vi "FisherPaykel GET Visa.vi"(8 "Error In":errorcluster) -> (0 "Error Out":errorcluster, 1 "Use GEA Inverter Output":bool, 2 "Disable Serial COM (Debug ONLY) OUT":bool, 3 "VISA Output":refnum<visa-resource-name>, 4 "Machine ID Output":string, 6 "Inverter ID Output":string)   [LabVIEW 2016]
uses:
  Trunk/Utility/LabVIEW GEA2 Toolkit v1.0.0.0/library/GEA2_Toolkit.lvlib
panel:
  in  "Tab Control":enum32{"F&P Inverter", "GEA Inverter", "Debug"}(tab)
  in  "Discover Motor Interfaces":bool
  out "Motor Controllers Found":refnum<visa-resource-name>[](array[refnum])
  in  "Motor Controller Reference":refnum<visa-resource-name>
  out "Message":string
  in  "Inverter ID":string(combo)
  in  "Machine ID":string(combo)
  out "Detected Green Beans":string[](array[string])
  in  "Use GEA Inverter":bool
  in  "Discover GE Interfaces":bool
  in  "Disable Serial COM (Debug ONLY)":bool
  in  "Complete":bool
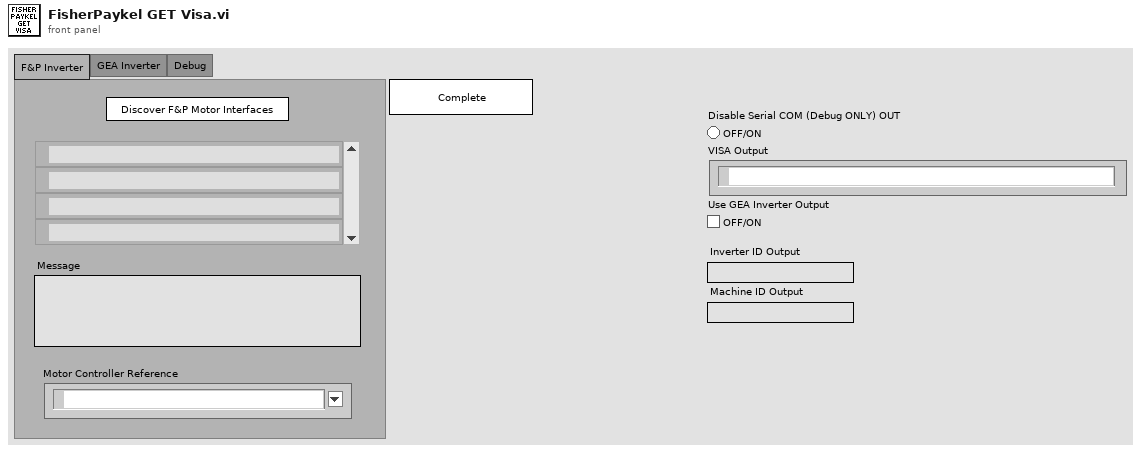
[diagram p1: front panel]
types:
  T1 = enum8{"Enabled", "Disabled", "Disabled and Grayed Out"}
  T2 = enum32{"invalid app kind", "Development System", "Run Time System", "Student Edition", "Embedded LabVIEW", "Evaluation", "Custom"}
  T3 = enum32{"Invalid", "Standard", "Closed", "Hidden", "Minimized", "Maximized"}
  T4 = cluster{"Core":cluster{"Current VI Reference":refnum<vi>, "Close Panel on Exit?":bool}, "Your Boolean data":bool, "Your string data":string}
  T5 = cluster{"Current VI Reference":refnum<vi>, "Close Panel on Exit?":bool}
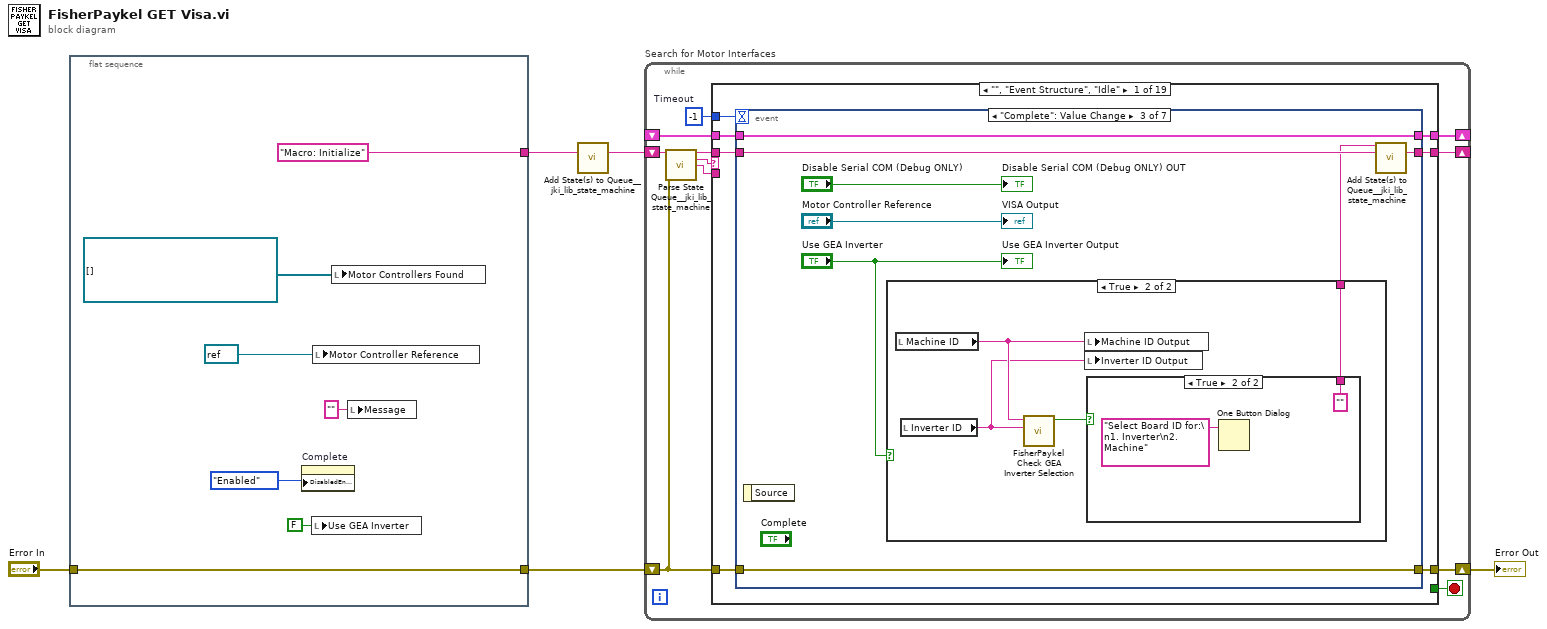
[diagram p0: block diagram]
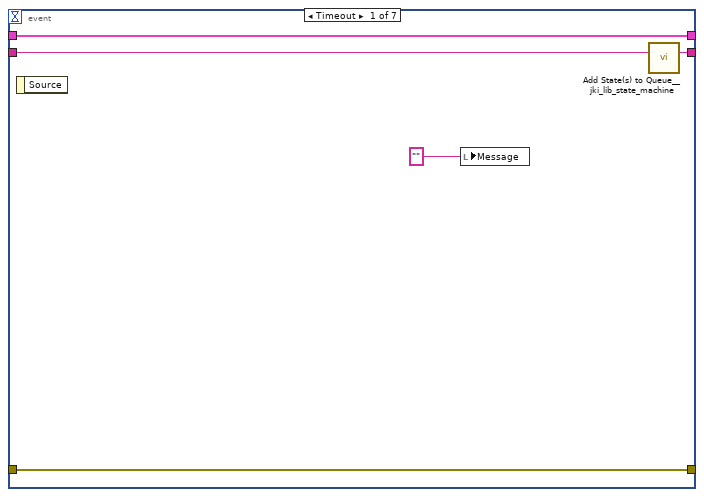
[diagram p2: hidden frame]
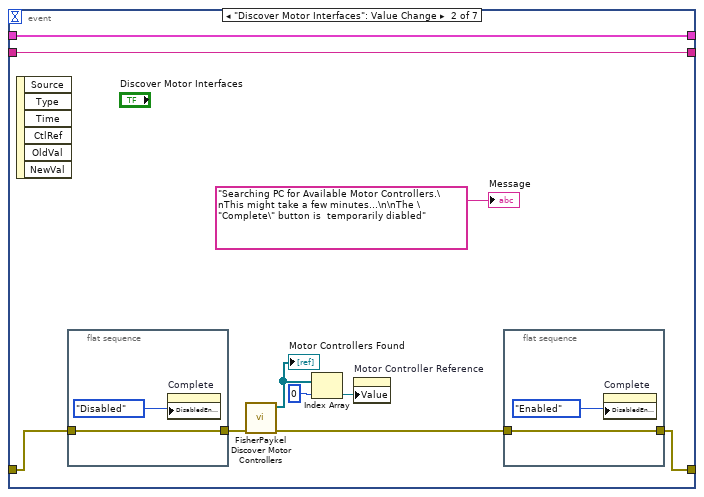
[diagram p3: hidden frame]
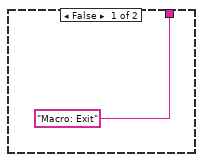
[diagram p4: hidden frame]
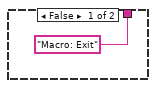
[diagram p5: hidden frame]
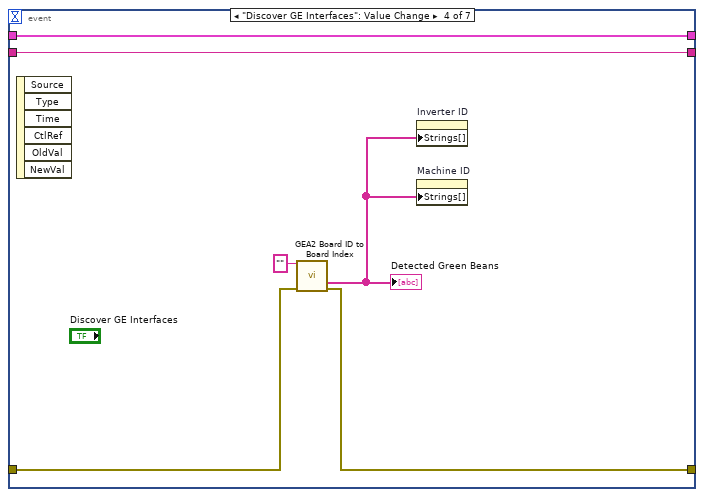
[diagram p6: hidden frame]
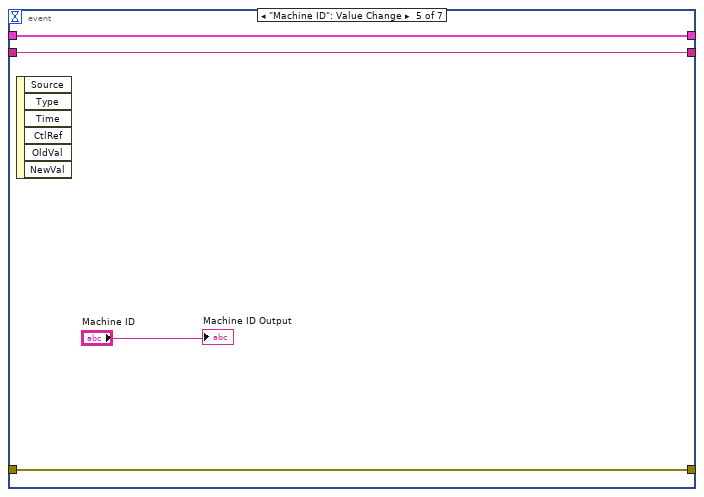
[diagram p7: hidden frame]
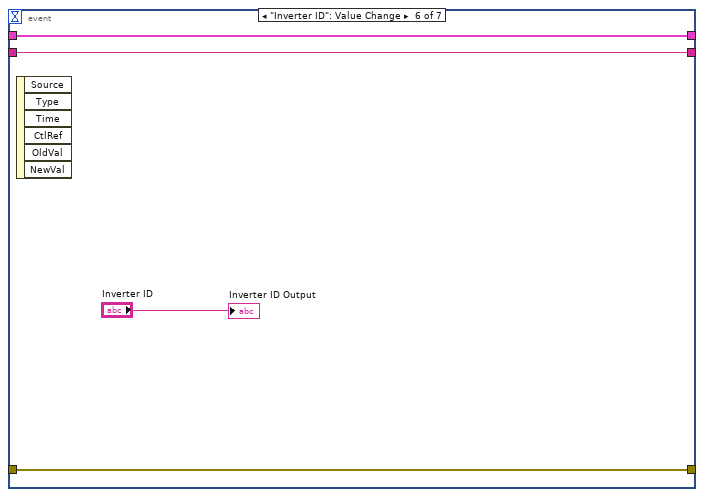
[diagram p8: hidden frame]
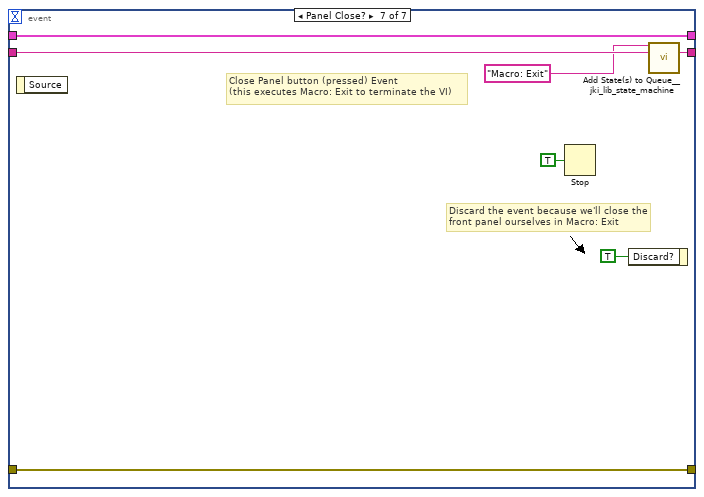
[diagram p9: hidden frame]
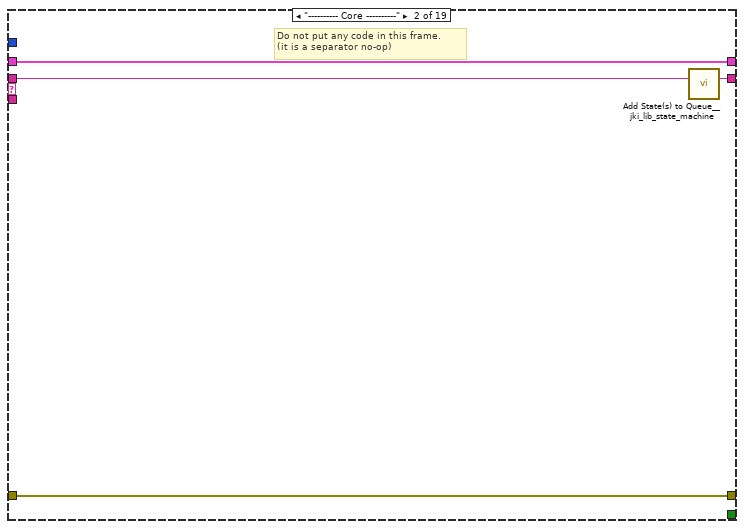
[diagram p10: hidden frame]
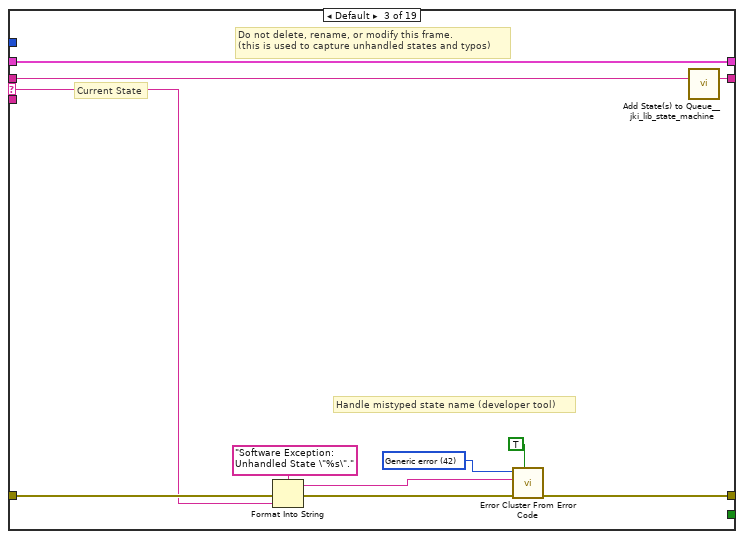
[diagram p11: hidden frame]
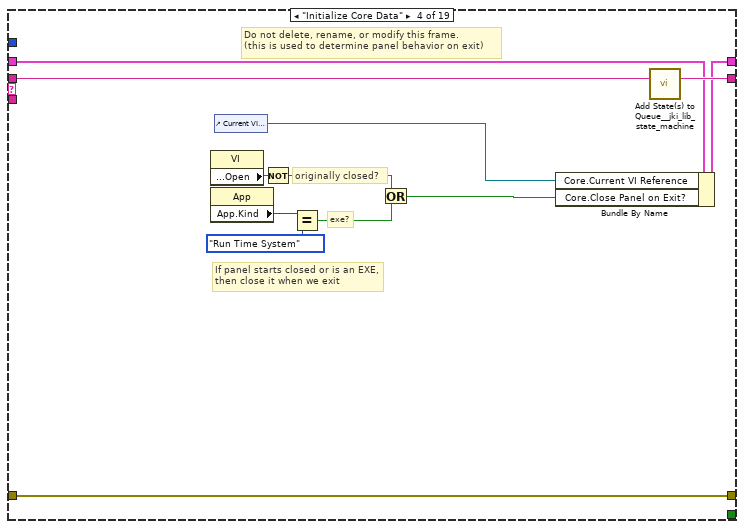
[diagram p12: hidden frame]
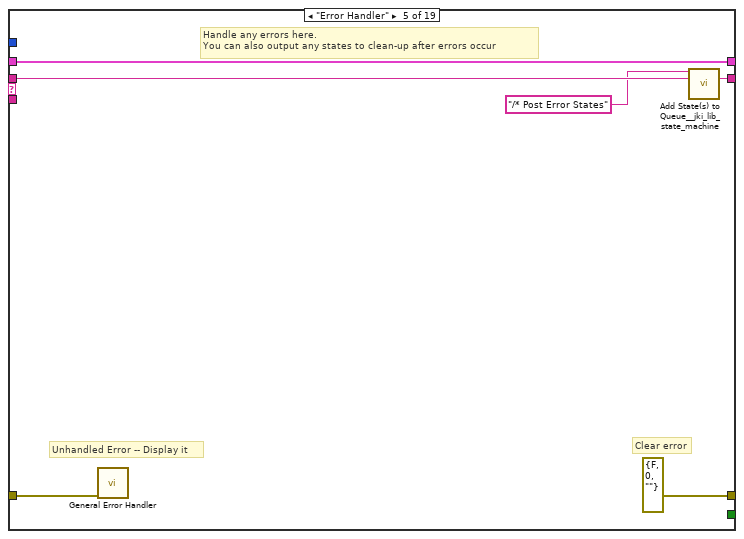
[diagram p13: hidden frame]
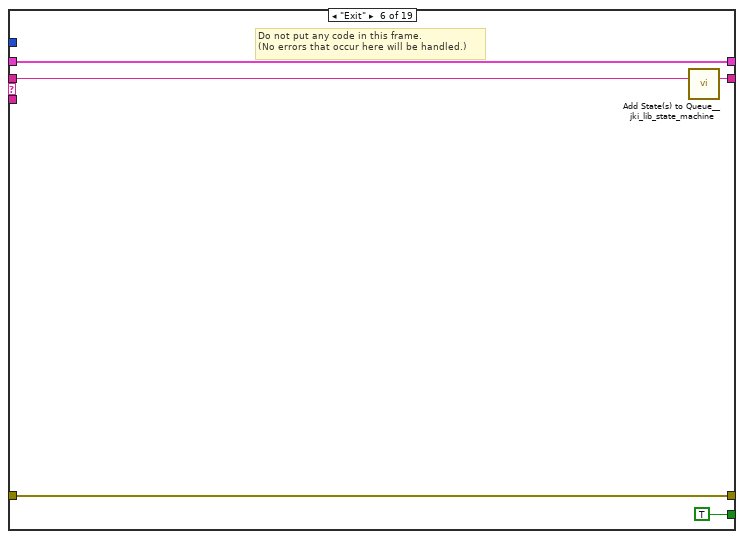
[diagram p14: hidden frame]
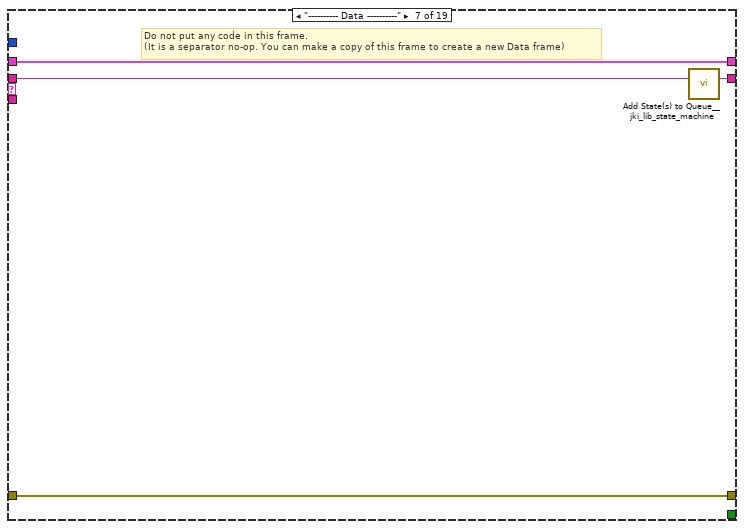
[diagram p15: hidden frame]
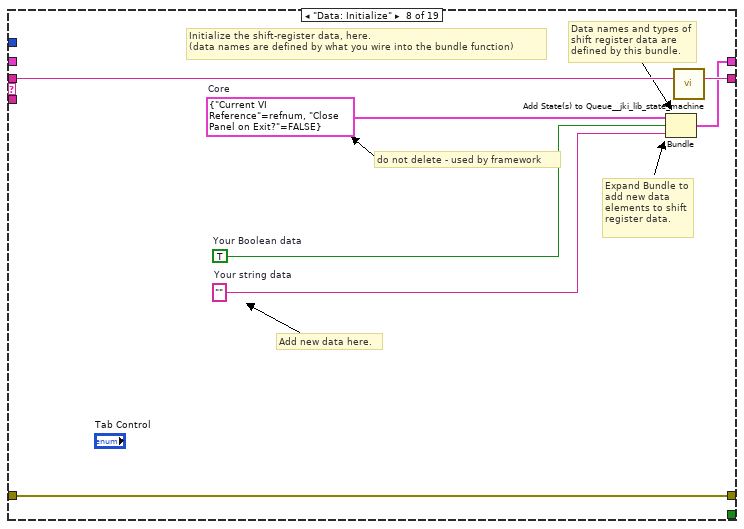
[diagram p16: hidden frame]
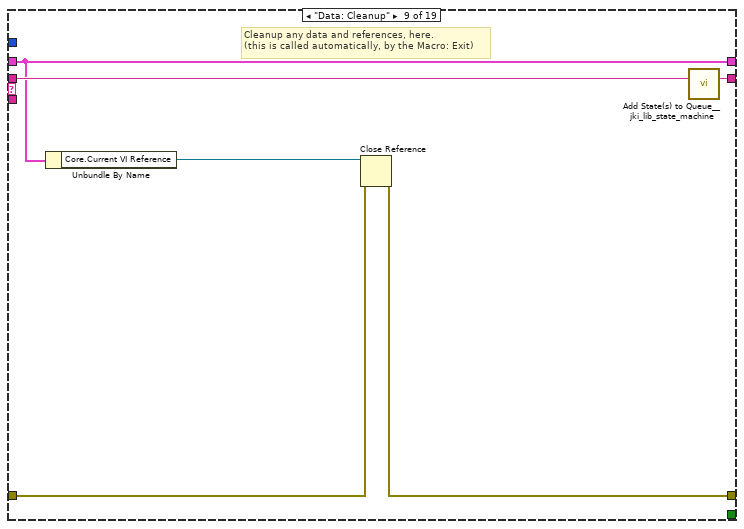
[diagram p17: hidden frame]
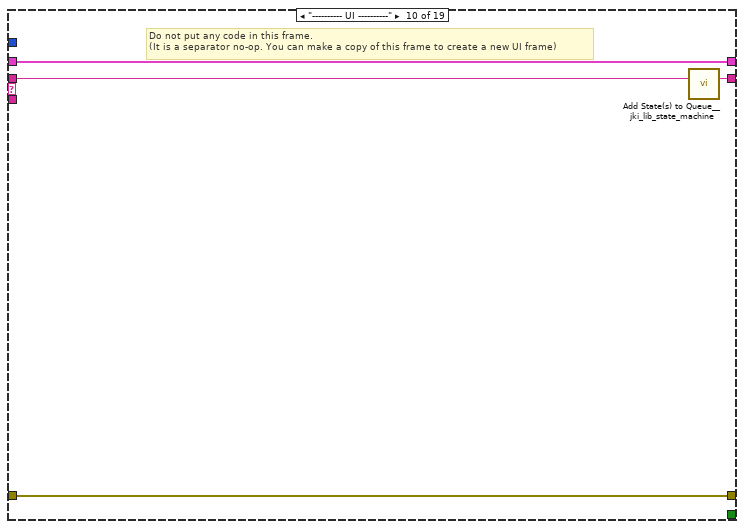
[diagram p18: hidden frame]
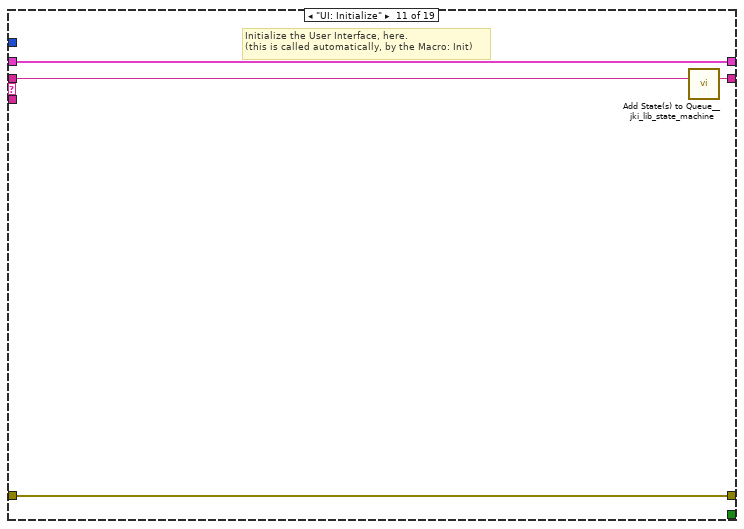
[diagram p19: hidden frame]
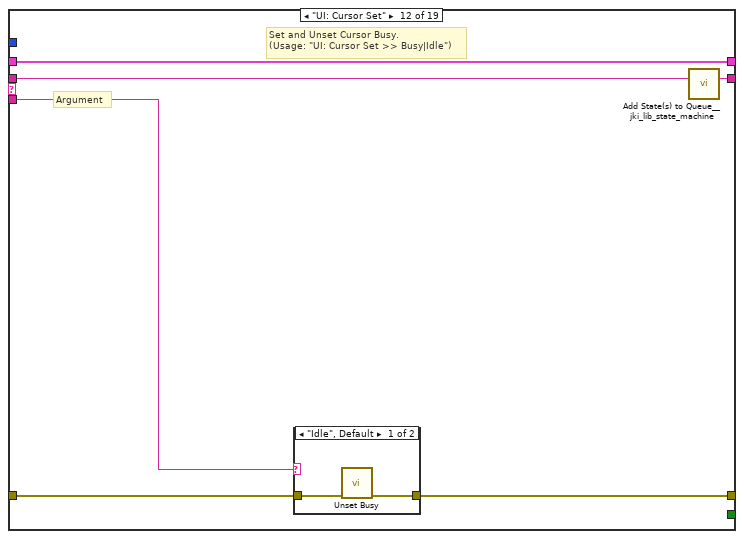
[diagram p20: hidden frame]
diagram:
  n1 = flat-sequence {
    tunnel: ["Macro: Initialize"] -> w4
    tunnel: [w7] -> w1
    tunnel: "Error In" -> [w7]
    frame #0 {
      n2 = property on="Complete" class="Bool"("DisabledEnum"=T1."Enabled" ("Disabled")) -> ()  [unwired: 2 in, 2 out]
      n3 = local write "Use GEA Inverter"(FALSE ("Use GEA Inverter")) -> ()
      n4 = local write "Motor Controller Reference"(refnum<visa-resource-name> refnum ("Motor Controller Reference")) -> ()
      n5 = local write "Motor Controllers Found"(refnum<visa-resource-name>[] [] ("Motor Controllers Found")) -> ()
      n6 = local write "Message"("" ("Message")) -> ()
    }
  }
  n7 = call <vilib>:"Add State(s) to Queue__jki_lib_state_machine.vi"("State(s) in (\"\")"=w4) -> ("States Out"=w5:string)  [unwired: 14 in]
  n8 = while "Search for Motor Interfaces" {
    shift-right: [w16] -> _
    shift-left: _ -> [w15]
    shift-right: [w19] -> w3
    shift-left: w1 -> [w13]
    shift-right: [w18] -> _
    shift-left: w5 -> [w20]
    stop <- w17 stop-if-true
    w14 = -1  # Timeout
    n9 = call <vilib>:"Parse State Queue__jki_lib_state_machine.vi"("State Queue"=w20, "Error In (no error)"=w13) -> ("Remaining States"=w22:string, "Current State"=w23:string, "Arguments"=w21:string)  [unwired: 11 in]
    n10 = case shown="\"\", \"Event Structure\", \"Idle\"" w23 {
      selector: w23 -> [_ _ w91 _ _ _ _ _ _ _ _ _ _ _ _ _ _ _ _]
      tunnel: w22 -> [w30 w90 w95 w113 w119 w124 w128 w135 w141 w145 w149 w155 w166 w192 w197 w207 w211 w215 w219]
      tunnel: w21 -> [_ _ _ _ _ _ _ _ _ _ _ w150 w160 _ _ _ _ _ _]
      tunnel: w15 -> [w28 w87 w93 w104 w116 w122 w125 _ w136 w142 w147 w153 w162 w189 w194 w204 w208 w212 w216]
      tunnel: [w27 w88 w97 w110 errorcluster {"status"=FALSE, "code"=0, "source"=""} ("error out") w121 w126 w132 w137 w143 w146 w151 w163 w190 w195 w205 w209 w213 w217] -> w19
      tunnel: w13 -> [w26 w88 w96 w110 w115 w121 w126 w132 w138 w143 w146 w152 w164 w190 w195 w205 w209 w213 w217]
      tunnel: [w29 w89 w94 w112 w118 w123 w127 w134 w140 w144 w148 w154 w165 w191 w196 w206 w210 w214 w218] -> w18
      tunnel: [_ _ _ _ _ TRUE _ _ _ _ _ _ _ _ _ _ _ _ _] -> w17
      tunnel: [w25 w87 w93 w111 w116 w122 w125 w133 w136 w142 w147 w153 w162 w189 w194 w204 w208 w212 w216] -> w16
      tunnel: w14 -> [w24 _ _ _ _ _ _ _ _ _ _ _ _ _ _ _ _ _ _]
      frame "", "Event Structure", "Idle" {
        n11 = event shown="[2] \"Complete\": Value Change" {
          selector: _ -> [_ _ _ _ _ _ _]
          dyn-events: _ -> [_ _ _ _ _ _ _]
          timeout: w24 -> [_ _ _ _ _ _ _]
          tunnel: w30 -> [w35 w41 w57 w68 w74 w78 w86]
          tunnel: [w34 w41 w56 w68 w74 w78 w85] -> w29
          tunnel: w28 -> [w33 w42 w54 w69 w75 w79 w83]
          tunnel: [w32 w36 w55 w70 w72 w76 w84] -> w27
          tunnel: w26 -> [w32 w39 w55 w71 w72 w76 w84]
          tunnel: [w33 w42 w54 w69 w75 w79 w83] -> w25
          event Timeout {
            n12 = event-data() -> ()  [unwired: 1 in, 1 out]
            n13 = local write "Message"("" ("Message")) -> ()
            n14 = call <vilib>:"Add State(s) to Queue__jki_lib_state_machine.vi"("State(s) in (\"\")"=w35) -> ("States Out"=w34:string)  [unwired: 14 in]
          }
          event "Discover Motor Interfaces": Value Change {
            n15 = event-data() -> ()  [unwired: 1 in, 6 out]
            n16 = flat-sequence {
              tunnel: w39 -> [w48]
              tunnel: [w48] -> w38
              frame #0 {
                n17 = property on="Complete" class="Bool"("DisabledEnum"=T1."Disabled" ("Disabled")) -> ()  [unwired: 2 in, 2 out]
              }
            }
            n18 = call "FisherPaykel Discover Motor Controllers.vi"("error in (no error)"=w38) -> ("Error Out"=w37:errorcluster, "Array"=w43:refnum<visa-resource-name>[])  [unwired: 9 in]
            "Motor Controllers Found" <- w43
            n19 = Index Array(array=w43, index=0) -> (element=w45:refnum<visa-resource-name>)
            n20 = property on="Motor Controller Reference" class="VISAName"("Value"=w45) -> ()  [unwired: 2 in, 2 out]
            n21 = flat-sequence {
              tunnel: w37 -> [w46]
              tunnel: [w46] -> w36
              frame #0 {
                n22 = property on="Complete" class="Bool"("DisabledEnum"=T1."Enabled" ("Disabled")) -> ()  [unwired: 2 in, 2 out]
              }
            }
            "Message" <- "Searching PC for Available Motor Controllers.\nThis might take a few minutes...\n\nThe \"Complete\" button is  temporarily diabled" ("Message")
          }
          event "Complete": Value Change {
            n23 = event-data() -> ()  [unwired: 1 in, 1 out]
            n24 = case shown="True" "Use GEA Inverter" {
              tunnel: ["Macro: Exit" w61] -> w50
              frame False {
              }
              frame True {
                n25 = local read "Machine ID"() -> (w60:string)
                n26 = local read "Inverter ID"() -> (w59:string)
                n27 = call "FisherPaykel Check GEA Inverter Selection.vi"("Inverter ID"=w59, "Machine ID"=w60) -> ("Throw Error?"=w62:bool)  [unwired: 8 in, 1 out]
                n28 = local write "Machine ID Output"(w60) -> ()
                n29 = local write "Inverter ID Output"(w59) -> ()
                n30 = case shown="True" w62 {
                  tunnel: ["Macro: Exit" ""] -> w61
                  frame False {
                  }
                  frame True {
                    n31 = One Button Dialog(message="Select Board ID for:\n1. Inverter\n2. Machine") -> ()  [unwired: 1 in, 1 out]
                  }
                }
              }
            }
            n32 = call <vilib>:"Add State(s) to Queue__jki_lib_state_machine.vi"("State(s) in Front (\"\")"=w50, "State(s) in (\"\")"=w57) -> ("States Out"=w56:string)  [unwired: 13 in]
            "VISA Output" <- "Motor Controller Reference"
            "Disable Serial COM (Debug ONLY) OUT" <- "Disable Serial COM (Debug ONLY)"
            "Use GEA Inverter Output" <- "Use GEA Inverter"
          }
          event "Discover GE Interfaces": Value Change {
            n33 = event-data() -> ()  [unwired: 1 in, 6 out]
            n34 = call "GEA2 Board ID to Board Index.vi"("Board ID"="", "Error In"=w71) -> ("Boards Found"=w66:string[], "Error Out"=w70:errorcluster)  [unwired: 9 in, 3 out]
            "Detected Green Beans" <- w66
            n35 = property on="Inverter ID" class="CmbBox"("Strings[]"=w66) -> ()  [unwired: 2 in, 2 out]
            n36 = property on="Machine ID" class="CmbBox"("Strings[]"=w66) -> ()  [unwired: 2 in, 2 out]
          }
          event "Machine ID": Value Change {
            n37 = event-data() -> ()  [unwired: 1 in, 6 out]
            "Machine ID Output" <- "Machine ID"
          }
          event "Inverter ID": Value Change {
            n38 = event-data() -> ()  [unwired: 1 in, 6 out]
            "Inverter ID Output" <- "Inverter ID"
          }
          event Panel Close? {
            # "Discard the event because we'll close the front panel ourselves in Macro: Exit"
            # "Close Panel button (pressed) Event\n(this executes Macro: Exit to terminate the VI)"
            n39 = event-data() -> ()  [unwired: 1 in, 1 out]
            n40 = Stop(stop? (T)=TRUE) -> ()
            n41 = event-data("Discard?"=TRUE) -> ()  [unwired: 1 in, 1 out]
            n42 = call <vilib>:"Add State(s) to Queue__jki_lib_state_machine.vi"("State(s) in Front (\"\")"="Macro: Exit", "State(s) in (\"\")"=w86) -> ("States Out"=w85:string)  [unwired: 13 in]
          }
        }
      }
      frame "---------- Core ----------" {
        # "Do not put any code in this frame.\n(it is a separator no-op)"
        n43 = call <vilib>:"Add State(s) to Queue__jki_lib_state_machine.vi"("State(s) in (\"\")"=w90) -> ("States Out"=w89:string)  [unwired: 14 in]
      }
      frame Default {
        w100 = 42 items=["No error", "Argument error", "Memory is full", "Out of zone", "End of file", "File already open", "Generic file I/O error", "File not found", "File permission error", "Disk is full", "Duplicate path", "Too many files open", "System feature not enabled", "Resource file not found", "Cannot add resource", "Resource not found", "Image not found", "Image memory error", "Pen does not exist", "Config type invalid", "Config token not found", "Config parse error", "Config memory error", "Bad external code format", "Bad external code offset", "External code not present", "Null window", "Destroy window error", "Null menu", "Print aborted", "Bad print record", "Print driver error", "Windows error during printing", "Memory error during printing", "Print dialog error", "Generic print error", "Invalid device refnum", "Device not found", "Device parameter error", "Device unit error", "Cannot open device", "Device call aborted", "Generic error", "Cancelled by user", "Object ID too low", "Object ID too high", "Object not in heap", "Unknown heap", "Unknown object (invalid DefProc)", "Unknown object (DefProc not in table)", "Message out of range", "Invalid (null) method", "Unknown message", "Manager call not supported", "Bad address", "Network operation in progress", "Network operation timed out", "Connection is busy", "Network attribute not supported", "Network error", "Address in use", "System out of memory", "Connection aborted", "Connection refused", "Not connected", "Already connected", "Connection closed", "Initialization error (interapplication manager)", "Bad occurrence", "Wait on unbound occurrence handler", "Occurrence queue overflow", "Datalog type conflict", "Unused", "Unrecognized type (interapplication manager)", "Memory corrupt", "Failed to make temporary DLL", "Old CIN version", "Drag socket not found", "Failed to load drop-object", "Failed to register OLE object", "Failed to release OLE object", "Format specifier type mismatch", "Unknown format specifier", "Too few format specifiers", "Too many format specifiers", "Scan failed", "Newer CIN version", "Error converting to variant", "Runtime menu error", "Password tampered", "Variant attribute not found", "Incompatible variant data type", "Event data is not available", "Event Store is not present", "Occurrence is not found", "Event Queue is not created", "Event info is not available", "Refnum passed is NULL", "Error retrieving Class GUID", "Error retrieving CoClass GUID", "Error retrieving TypeLib GUID.", "Bad built application magic bytes.", "Specific driver is different from the specific driver associated with the Logical Name.", "There is no session opened to the class driver.", "Max Error", "MAX - Error with config objects", "MAX - Error loading configuration", "MAX - Group not supported"]
        # "Current State"
        # "Do not delete, rename, or modify this frame.\n(this is used to capture unhandled states and typos)"
        # "Handle mistyped state name (developer tool)"
        n44 = Format Into String(format string="Software Exception: Unhandled State \"%s\"." ("message"), error in=w96, w91) -> (resulting string=w99:string, error out=w98:errorcluster)  [unwired: 1 in]
        n45 = call <vilib>:"Error Cluster From Error Code.vi"("show call chain? (False)"=TRUE, "error in (no error)"=w98, "error message (\"\")"=w99, "error code (0)"=w100) -> ("error out"=w97:errorcluster)  [unwired: 5 in]
        n46 = call <vilib>:"Add State(s) to Queue__jki_lib_state_machine.vi"("State(s) in (\"\")"=w95) -> ("States Out"=w94:string)  [unwired: 14 in]
      }
      frame "Initialize Core Data" {
        # "Do not delete, rename, or modify this frame.\n(this is used to determine panel behavior on exit)"
        # "originally closed?"
        # "exe?"
        # "If panel starts closed or is an EXE, then close it when we exit"
        n47 = property class="VI"() -> ("Front Panel.Open"=w109:bool)  [unwired: 2 in, 2 out]
        n48 = property class="App"() -> ("App.Kind"=w108:T2)  [unwired: 2 in, 2 out]
        n49 = control-ref of="Current VI Reference"() -> (w102:refnum<vi>)
        n50 = Not(x=w109) -> (.not. x?=w106:bool)
        n51 = Equal?(x=w108, y=T2."Run Time System" ("Application:Kind")) -> (x = y?=w105:bool)
        n52 = Or(x=w106, y=w105) -> (x .or. y?=w103:bool)
        n53 = Bundle By Name(cluster=w104, "Core.Current VI Reference"=w102, "Core.Close Panel on Exit?"=w103) -> (w111:T4)
        n54 = call <vilib>:"Add State(s) to Queue__jki_lib_state_machine.vi"("State(s) in (\"\")"=w113) -> ("States Out"=w112:string)  [unwired: 14 in]
      }
      frame "Error Handler" {
        # "Unhandled Error -- Display it"
        # "Handle any errors here.\nYou can also output any states to clean-up after errors occur"
        # "Clear error"
        n55 = call <vilib>:"General Error Handler.vi"("error in (no error)"=w115) -> ()  [unwired: 10 in, 5 out]
        n56 = call <vilib>:"Add State(s) to Queue__jki_lib_state_machine.vi"("State(s) in Front (\"\")"="/* Post Error States", "State(s) in (\"\")"=w119) -> ("States Out"=w118:string)  [unwired: 13 in]
      }
      frame "Exit" {
        # "Do not put any code in this frame.\n(No errors that occur here will be handled.)"
        n57 = call <vilib>:"Add State(s) to Queue__jki_lib_state_machine.vi"("State(s) in (\"\")"=w124) -> ("States Out"=w123:string)  [unwired: 14 in]
      }
      frame "---------- Data ----------" {
        # "Do not put any code in this frame.\n(It is a separator no-op. You can make a copy of this frame to create a new Data frame)"
        n58 = call <vilib>:"Add State(s) to Queue__jki_lib_state_machine.vi"("State(s) in (\"\")"=w128) -> ("States Out"=w127:string)  [unwired: 14 in]
      }
      frame "Data: Initialize" {
        w129 = T5 {"Current VI Reference"=refnum, "Close Panel on Exit?"=FALSE}  # Core
        w131 = TRUE  # Your Boolean data
        w130 = ""  # Your string data
        # "do not delete - used by framework"
        # "Expand Bundle to add new data elements to shift register data."
        # "Add new data here."
        # "Data names and types of shift register data are defined by this bundle."
        # "Initialize the shift-register data, here.\n(data names are defined by what you wire into the bundle function)"
        n59 = Bundle("Core"=w129, "Your Boolean data"=w131, "Your string data"=w130) -> (w133:T4)  [unwired: 1 in]
        n60 = call <vilib>:"Add State(s) to Queue__jki_lib_state_machine.vi"("State(s) in (\"\")"=w135) -> ("States Out"=w134:string)  [unwired: 14 in]
      }
      frame "Data: Cleanup" {
        # "Cleanup any data and references, here.\n(this is called automatically, by the Macro: Exit)"
        n61 = Unbundle By Name(w136) -> ("Core.Current VI Reference"=w139:refnum<vi>)
        n62 = Close Reference(reference=w139, error in (no error)=w138) -> (error out=w137:errorcluster)
        n63 = call <vilib>:"Add State(s) to Queue__jki_lib_state_machine.vi"("State(s) in (\"\")"=w141) -> ("States Out"=w140:string)  [unwired: 14 in]
      }
      frame "---------- UI ----------" {
        # "Do not put any code in this frame.\n(It is a separator no-op. You can make a copy of this frame to create a new UI frame)"
        n64 = call <vilib>:"Add State(s) to Queue__jki_lib_state_machine.vi"("State(s) in (\"\")"=w145) -> ("States Out"=w144:string)  [unwired: 14 in]
      }
      frame "UI: Initialize" {
        # "Initialize the User Interface, here.\n(this is called automatically, by the Macro: Init)"
        n65 = call <vilib>:"Add State(s) to Queue__jki_lib_state_machine.vi"("State(s) in (\"\")"=w149) -> ("States Out"=w148:string)  [unwired: 14 in]
      }
      frame "UI: Cursor Set" {
        # "Argument"
        # "Set and Unset Cursor Busy.\n(Usage: \"UI: Cursor Set >> Busy|Idle\")"
        n66 = case shown="\"Idle\", Default" w150 {
          tunnel: w152 -> [w157 w159]
          tunnel: [w156 w158] -> w151
          frame "Idle", Default {
            n67 = call <vilib>:"Unset Busy.vi"("error in (no error)"=w157) -> ("error out"=w156:errorcluster)  [unwired: 10 in]
          }
          frame "Busy" {
            n68 = call <vilib>:"Set Busy.vi"("error in (no error)"=w159) -> ("error out"=w158:errorcluster)  [unwired: 9 in, 1 out]
          }
        }
        n69 = call <vilib>:"Add State(s) to Queue__jki_lib_state_machine.vi"("State(s) in (\"\")"=w155) -> ("States Out"=w154:string)  [unwired: 14 in]
      }
      frame "UI: Front Panel State" {
        # "Argument"
        # "Set Front Panel Open or Closed\n(Usage: \"UI: Front Panel State >> Open|Close\")"
        n70 = Unbundle By Name(w162) -> ("Core.Current VI Reference"=w161:refnum<vi>)
        n71 = case shown="\"Open\", Default" w160 {
          tunnel: w164 -> [w170 w183]
          tunnel: [w172 w184] -> w163
          tunnel: w161 -> [w171 w181]
          frame "Open", Default {
            n72 = property class="VI"(reference=w171, error in=w170) -> (reference out=w168:refnum<vi>, error out=w169:errorcluster, "Front Panel.Open"=w167:bool)
            n73 = case shown="False" w167 {
              tunnel: [w175 w178] -> w172
              tunnel: w169 -> [w174 w178]
              tunnel: w168 -> [w173 _]
              frame False {
                n74 = invoke class="VI" method="FP.Open"(reference=w173, error in=w174, "Activate"=TRUE, "State"=T3."Standard") -> (error out=w175:errorcluster)  [unwired: 1 in, 4 out]
              }
              frame True {
              }
            }
          }
          frame "Close" {
            n75 = property class="VI"(reference=w181, error in=w183) -> (reference out=w180:refnum<vi>, error out=w182:errorcluster, "Front Panel.Open"=w179:bool)
            n76 = case shown="True" w179 {
              tunnel: [w185 w188] -> w184
              tunnel: w182 -> [w185 w187]
              tunnel: w180 -> [_ w186]
              frame False {
              }
              frame True {
                n77 = invoke class="VI" method="FP.Close"(reference=w186, error in=w187) -> (error out=w188:errorcluster)  [unwired: 1 in, 2 out]
              }
            }
          }
        }
        n78 = call <vilib>:"Add State(s) to Queue__jki_lib_state_machine.vi"("State(s) in (\"\")"=w166) -> ("States Out"=w165:string)  [unwired: 14 in]
      }
      frame "---------- Macro ----------" {
        # "Do not put any code in this frame.\n(It is a separator no-op. You can make a copy of this frame to create a new Macro frame)"
        n79 = call <vilib>:"Add State(s) to Queue__jki_lib_state_machine.vi"("State(s) in (\"\")"=w192) -> ("States Out"=w191:string)  [unwired: 14 in]
      }
      frame "Macro: Initialize" {
        w193 = "Data: Initialize\nInitialize Core Data\nUI: Initialize\nUI: Front Panel State >> Open"  # Data: Initialize Initialize Core Data UI: Initialize UI: Front Panel State >> Open
        # "Initialization Macro\n(This is called once, when the VI starts)"
        n80 = call <vilib>:"Add State(s) to Queue__jki_lib_state_machine.vi"("State(s) in Front (\"\")"=w193, "State(s) in (\"\")"=w197) -> ("States Out"=w196:string)  [unwired: 13 in]
      }
      frame "Macro: Exit" {
        # "Exit Macro\n(This is called once, when the VI exits)"
        n81 = Unbundle By Name(w204) -> ("Core.Close Panel on Exit?"=w203:bool)
        n82 = Select(t="UI: Front Panel State >> Close", s=w203, f="") -> (s? t:f=w200:string)
        n83 = call <vilib>:"Add State(s) to Queue__jki_lib_state_machine.vi"("State(s) in (\"\")"=w200, "State(s) at Back (\"\")"="Data: Cleanup\nExit") -> ("States Out"=w198:string)  [unwired: 13 in]
        n84 = call <vilib>:"Add State(s) to Queue__jki_lib_state_machine.vi"("State(s) in Front (\"\")"=w198, "State(s) in (\"\")"=w207) -> ("States Out"=w206:string)  [unwired: 13 in]
      }
      frame "---------- New Category ----------" {
        # "Template Separator\n(You can make a copy of, or modify, this frame)"
        n85 = call <vilib>:"Add State(s) to Queue__jki_lib_state_machine.vi"("State(s) in (\"\")"=w211) -> ("States Out"=w210:string)  [unwired: 14 in]
      }
      frame "New Category: 1" {
        # "Your code here.\n(You can make a copy of, or modify, this frame)"
        n86 = call <vilib>:"Add State(s) to Queue__jki_lib_state_machine.vi"("State(s) in (\"\")"=w215) -> ("States Out"=w214:string)  [unwired: 14 in]
      }
      frame "New Category: 2" {
        # "Your code here.\n(You can make a copy of, or modify, this frame)"
        n87 = call <vilib>:"Add State(s) to Queue__jki_lib_state_machine.vi"("State(s) in (\"\")"=w219) -> ("States Out"=w218:string)  [unwired: 14 in]
      }
    }
  }
  "Error Out" <- w3
